vi "Suggest New Attribute ID.vi"() -> ()   [LabVIEW 2023]
panel:
  in  "Manual":bool
  out "Calc Meas ID End":u32 format="%.0x"
  out "Array 2":u32[](array[numeric]) format="%.0x"
  in  "Meas ID End":u32=1114112 format="%.0x"
  in  "Meas ID Start":u32=1110016 format="%.0x"
  out "Array":u32[](array[numeric]) format="%.0x"
  out "error out":errorcluster
  out "Number of IDs found":i32
  out "Last ID used":string
  out "Suggested New ID":string
  in  "file path":path=path "E:/Dev/ni-central/src/rfmx/SpecAn/RFmxSpecAnLV/source/resource/objmgr/RFmxSpecAnAttributes.xml"
  # "Select the attributes xml file path and run the program"
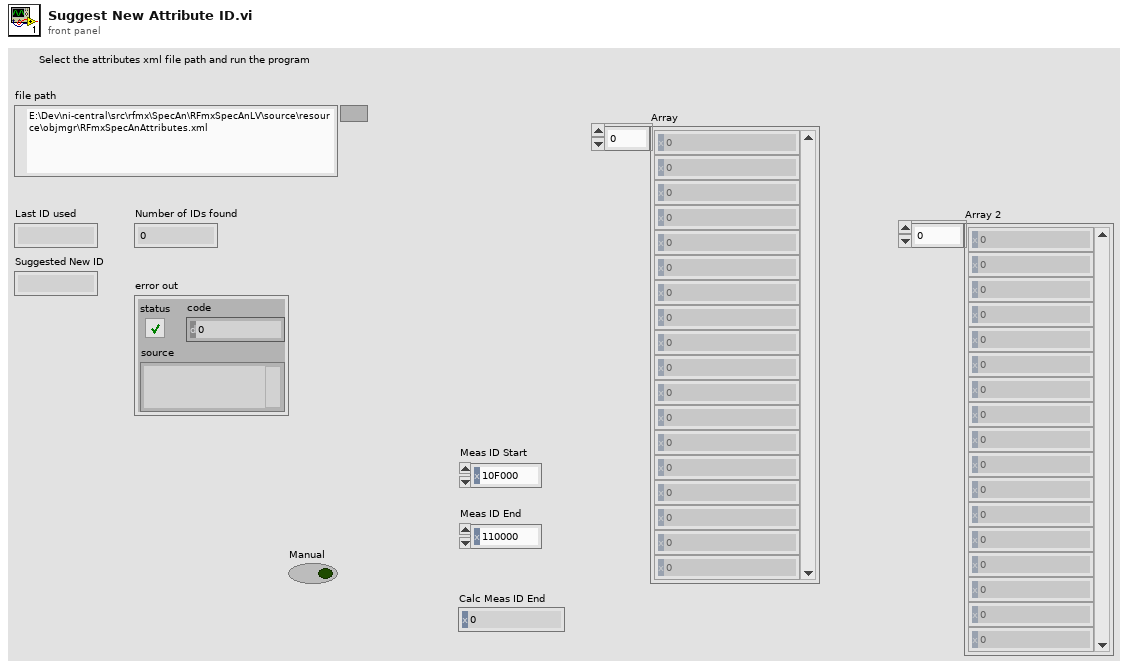
[diagram p1: front panel]
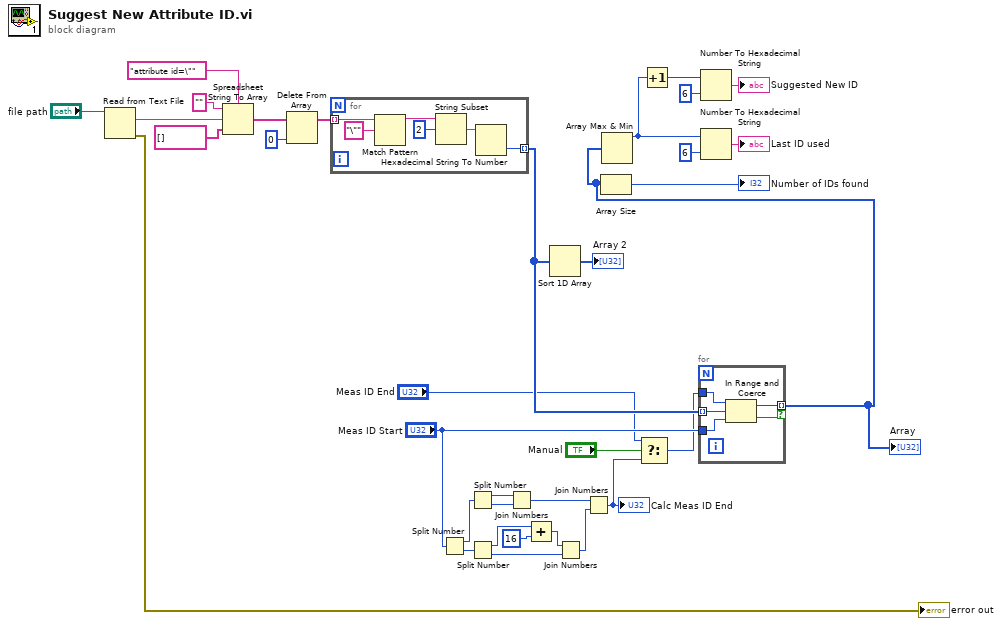
[diagram p0: block diagram]
diagram:
  n1 = Read from Text File(file (use dialog)="file path") -> (text=w26:string, error out=→"error out":errorcluster)  [unwired: 3 in, 2 out]
  n2 = Spreadsheet String To Array(delimiter (Tab)="attribute id=\"" ("regular expression"), format string="", spreadsheet string=w26, array type (2D Dbl)=string[] [] ("format string")) -> (array=w24:string[])
  n3 = Delete From Array(array=w24, index=0) -> (array with subset deleted=w23:string[])  [unwired: 1 in, 1 out]
  n4 = for {
    tunnel: w23 -> [w40] mode=indexing
    tunnel: [w37] -> w17 mode=indexing
    n5 = Match Pattern(string=w40, regular expression="\"") -> (before substring=w35:string)  [unwired: 1 in, 3 out]
    n6 = String Subset(string=w35, offset (0)=2) -> (substring=w36:string)  [unwired: 1 in]
    n7 = Hexadecimal String To Number(string=w36) -> (number=w37:u32)  [unwired: 2 in, 1 out]
  }
  n8 = Split Number(x="Meas ID Start") -> (hi(x)=w13:u16, lo(x)=w15:u16)
  n9 = Split Number(x=w13) -> (hi(x)=w11:u8, lo(x)=w10:u8)
  n10 = Split Number(x=w15) -> (hi(x)=w14:u8, lo(x)=w8:u8)
  n11 = Join Numbers(hi=w11, lo=w10) -> ((hi.lo)=w6:u16)
  n12 = Add(x=w14, y=u8 16) -> (x+y=w9:u8)
  n13 = Sort 1D Array(array=w17) -> (sorted array=→"Array 2":u32[])
  n14 = Join Numbers(hi=w9, lo=w8) -> ((hi.lo)=w7:u16)
  n15 = Join Numbers(hi=w6, lo=w7) -> ((hi.lo)=w4:u32)
  "Calc Meas ID End" <- w4
  n16 = Select(t="Meas ID End", s="Manual", f=w4) -> (s? t:f=w2:u32)
  n17 = for {
    tunnel: "Meas ID Start" -> [w42]
    tunnel: w17 -> [w45] mode=indexing
    tunnel: w2 -> [w41]
    tunnel: [w44] -> w18 mode=indexing if=w43
    n18 = In Range and Coerce(upper limit=w41, x=w45, lower limit=w42) -> (coerced(x)=w44:u32, In Range?=w43:bool)
  }
  "Array" <- w18
  n19 = Array Size(array=w18) -> (size(s)=→"Number of IDs found":i32)
  n20 = Array Max & Min(array=w18) -> (max value=w29:u32)  [unwired: 3 out]
  n21 = Increment(x=w29) -> (x+1=w34:u32)
  n22 = Number To Hexadecimal String(1:i16 6 ("width (-)"), 2:w34) -> (0:→"Suggested New ID":string)
  n23 = Number To Hexadecimal String(1:i16 6 ("width (-)"), 2:w29) -> (0:→"Last ID used":string)
